vi "Wektor zapisu.vi"(0 "Rzeczywiste f [Hz]":dbl[](array[numeric]), 1 "Prêdkoœæ zmierzona":dbl, 5 "Obliczone Amplitudy[dB]":dbl[](array[numeric]), 9 "Rzeczywiste fp [Hz]":dbl[](array[numeric]), 11 "Obliczone Amplitudy_fp [dB]":dbl[](array[numeric]), 12 "Poœlizg":dbl, 13 "Liczba prêtów":dbl) -> (8 "Wyjœcie":dbl[](array[numeric]))   [LabVIEW 2018]
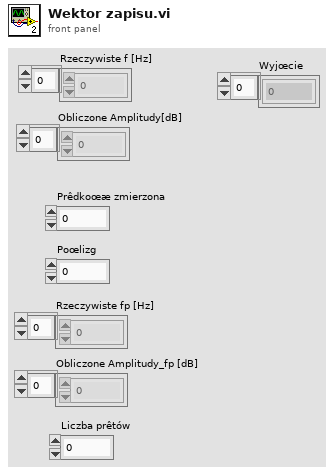
[diagram p1: front panel]
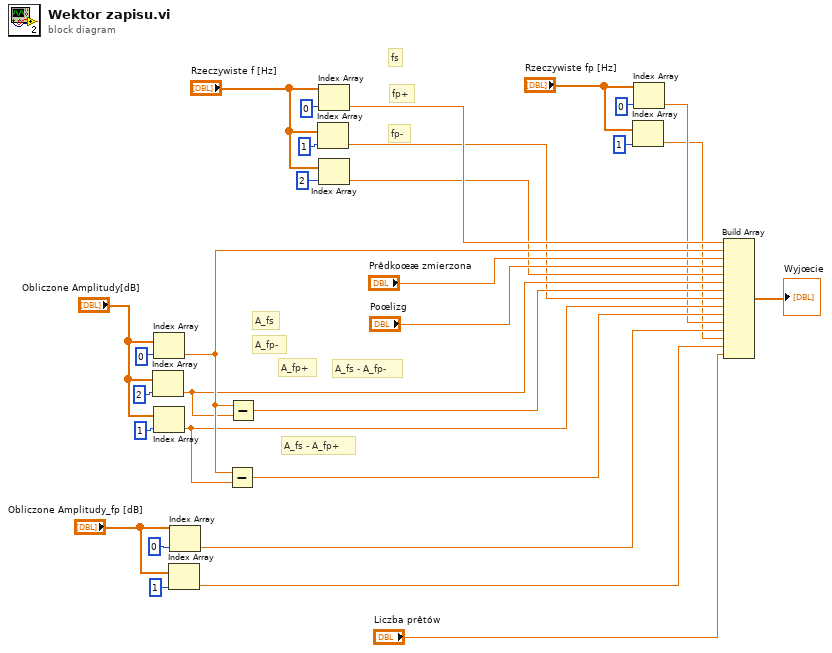
[diagram p0: block diagram]
diagram:
  # "fp-"
  # "fp+"
  # "fs"
  # "A_fs - A_fp-"
  # "A_fs - A_fp+"
  # "A_fp+"
  # "A_fs"
  # "A_fp-"
  n1 = Index Array(array="Obliczone Amplitudy[dB]", index=2) -> (element=w13:dbl)
  n2 = Index Array(array="Obliczone Amplitudy[dB]", index=0) -> (element=w17:dbl)
  n3 = Index Array(array="Obliczone Amplitudy[dB]", index=1) -> (element=w10:dbl)
  n4 = Index Array(array="Obliczone Amplitudy_fp [dB]", index=1) -> (element=w5:dbl)
  n5 = Index Array(array="Obliczone Amplitudy_fp [dB]", index=0) -> (element=w7:dbl)
  n6 = Subtract(x=w17, y=w10) -> (x-y=w9:dbl)
  n7 = Subtract(x=w17, y=w13) -> (x-y=w12:dbl)
  n8 = Index Array(array="Rzeczywiste f [Hz]", index=1) -> (element=w11:dbl)
  n9 = Index Array(array="Rzeczywiste f [Hz]", index=0) -> (element=w18:dbl)
  n10 = Index Array(array="Rzeczywiste f [Hz]", index=2) -> (element=w14:dbl)
  n11 = Index Array(array="Rzeczywiste fp [Hz]", index=1) -> (element=w6:dbl)
  n12 = Index Array(array="Rzeczywiste fp [Hz]", index=0) -> (element=w8:dbl)
  n13 = Build Array(w18, w17, "Prêdkoœæ zmierzona", "Poœlizg", w14, w13, w12, w11, w10, w9, w8, w7, w6, w5, "Liczba prêtów") -> (→"Wyjœcie":dbl[])
